vi "AFMss_control_DelayObserver_trajTrack.vi"() -> ()   [LabVIEW 2017]
uses:
  controls/controlParams_tracktraj.ctl
  controls/Xdelay.ctl
  <vilib>/rvi/Emulation/niFpgaGetClockAttributes.vi
  <vilib>/rvi/Emulation/niFpgaSctlEmulationGetInTimedLoop.vi
  <vilib>/rvi/Emulation/niFpgaEmulationReportErrorSimple.vi
  <vilib>/rvi/eio/common/nirviEmuTemplateMethod_errors.vi
  <vilib>/rvi/Emulation/niFpgaCriticalErrorInLSC.vi
  <vilib>/rvi/DataTransferAndStorage/Container/Common/niFpgaContainerExecOnDevCompGetState.vi
  <vilib>/rvi/Emulation/niFpgaEmulationIsFPGAContextNoSignature.vi
  <vilib>/rvi/DataTransferAndStorage/Container/Common/niFpgaContainerGetUniqueNameForEmu.vi
  <vilib>/rvi/Memory/Memory_Emulation/niFpgaMemoryEmulationCacheClearOnFirstRun.vi
  <vilib>/rvi/Memory/Memory_Emulation/nirvimemoryEmulationManagerCache_MakeExclusive.vi
  <vilib>/rvi/Memory/Memory_Emulation/niFpgaMemoryEmulationValidateCache.vi
  <vilib>/rvi/Memory/Memory_Emulation/nirvimemoryEmulationManagerCache_InsertValue.vi
  <vilib>/Utility/error.llb/Clear Errors.vi
  <vilib>/rvi/Memory/Memory_Emulation/nirvimemoryEmulationManagerCache_ReleaseExclusive.vi
  <vilib>/rvi/Memory/Memory_Emulation/nirvimemoryEmulationManagerCache_GetValue.vi
  <vilib>/rvi/Memory/Memory_Emulation/nirvimemoryEmulationManagerCache_SetValue.vi
  <vilib>/rvi/Emulation/niFpgaProcessEmulError.vi
  <vilib>/rvi/interface/RandomDataEmulation/niFpgaRandomDataHandleErrors.vi
  <vilib>/eio/EIONode/EIONode.xnode
  <vilib>/rvi/DataTransferAndStorage/Container/XNode/niFpgaContainer.xnode
  <vilib>/rvi/DataTransferAndStorage/Register/Emulation/niFpgaRegisterEmulationRefIn.vi
  <vilib>/rvi/interface/RandomDataEmulation/nirviRandomDataFpgaReadWriteTemplate.vi
  <vilib>/rvi/FXPMathLib/FxpSub/XNode/nifxpmath_Sub.xnode
  <vilib>/rvi/FXPMathLib/sim/FxpSim.dll
panel:
  out "Xd_out(k+1)":T1
  out "yk":sgl
  out "u_xk":sgl
  out "yuxk TO":bool
  out "YK TO":bool
  out "UK TO":bool
  in  "Cluster":T2={"umax"=3.0, "y_ref(k)"=0.0, "Ki"=0.0, "y(k) (from plant)"=0.0, "ND"=0, "NS"=0, "u_Kx_ref(k)"=0.0} {"u_Kx_ref(k)" format="%#_13g"; "Ki" format="%#_13g"; "y_ref(k)" format="%#_13g"; "umax" format="%#_13g"}
  out "Unstable Traj":bool
  out "ND":i16=2
  out "Loop Done":bool
  in  "Settle Ticks":i16=1000
  in  "False  = cont run":bool=TRUE
  in  "Abort":bool=TRUE
  in  "iters":i16=1
  in  "ymax":sgl=4.0 format="%#_13g"
  in  "TsTicks":i16
  out "Loop Ticks (benchmark)":i16
  out "NS":i16=2
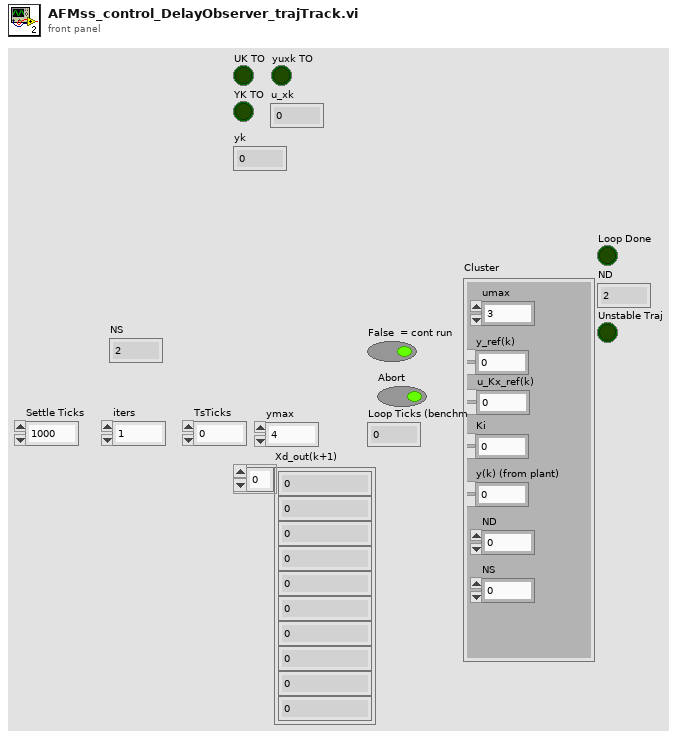
[diagram p1: front panel]
types:
  T1 = typedef "Xdelay.ctl" = sgl[]
  T2 = typedef "controlParams_tracktraj.ctl" = cluster{"umax":sgl, "y_ref(k)":sgl, "Ki":sgl, "y(k) (from plant)":sgl, "ND":i16, "NS":i16, "u_Kx_ref(k)":sgl}
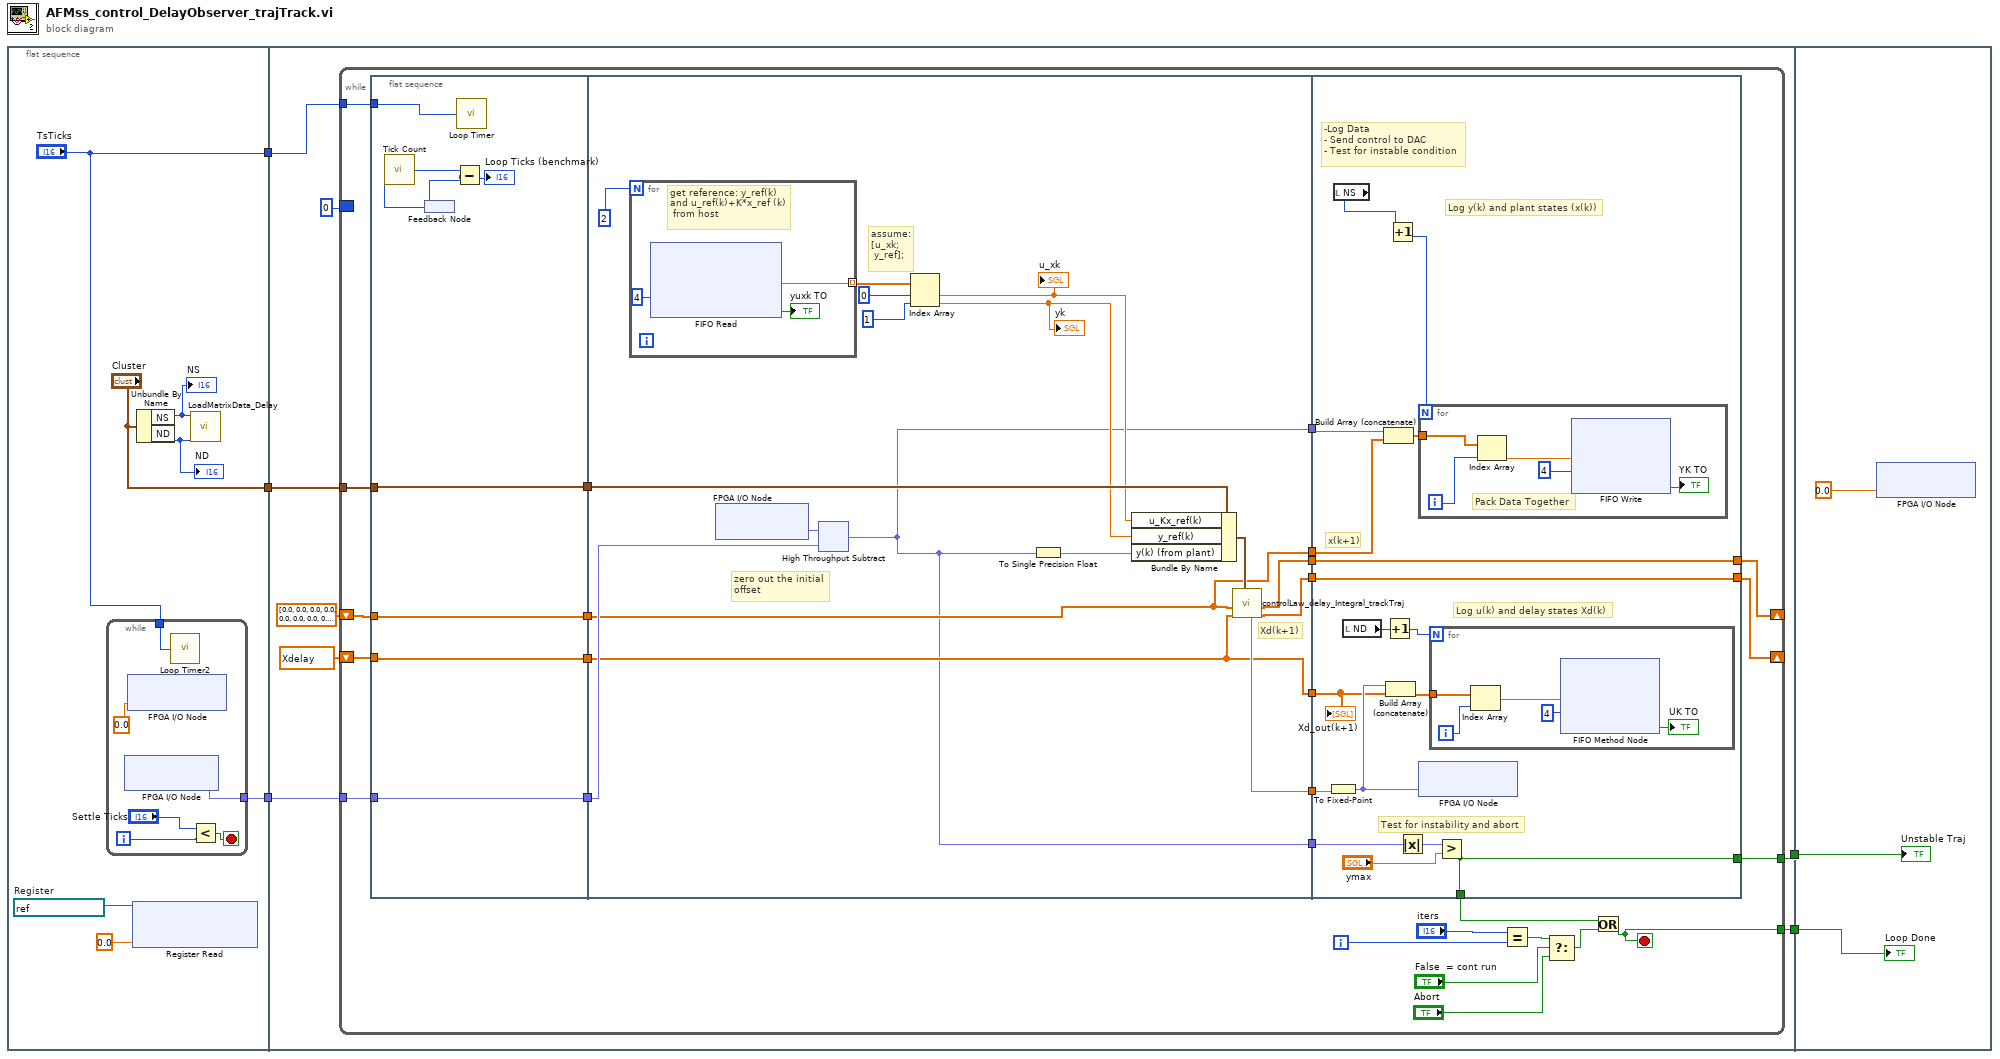
[diagram p0: block diagram]
diagram:
  n1 = flat-sequence {
    tunnel: ["TsTicks"] -> w5
    tunnel: [w12] -> w4
    tunnel: ["Cluster"] -> w2
    tunnel: w5 -> [w25]
    tunnel: w4 -> [w24]
    tunnel: [w21] -> w3
    tunnel: w2 -> [w20]
    tunnel: [w19] -> w1
    tunnel: w3 -> [w110]
    tunnel: w1 -> [w109]
    frame #0 {
      w10 = refnum<k21> "accumulator"  # Register
      # "Load Matrix Data"
      n2 = while {
        tunnel: [w18] -> w12
        tunnel: "TsTicks" -> [w17]
        i -> [w13]
        stop <- w15 stop-if-true
        n3 = xnode "FPGA I/O Node"() -> ("Mod2/AI0"=w18:fxp<+/-,24,5>)  [unwired: 1 in, 1 out]
        n4 = xnode "FPGA I/O Node"("Mod1/AO0"=sgl 0.0) -> ()  [unwired: 1 in, 1 out]
        n5 = call "Loop Timer2"("Count(Ticks)"=w17) -> ()  [unwired: 1 out]
        n6 = Less?(x="Settle Ticks", y=w13) -> (x < y?=w15:bool)
      }
      n7 = xnode ("Register Read")("Data"=sgl 0.0, "Register In"=w10) -> ()  [unwired: 1 out]
      n8 = Unbundle By Name("Cluster") -> ("NS"=w8:i16, "ND"=w7:i16)
      "NS" <- w8
      "ND" <- w7
      n9 = call "LoadMatrixData_Delay.vi"("Nd"=w7, "NS"=w8) -> ()  [unwired: 9 in, 1 out]
    }
    frame #1 {
      n10 = while {
        border: i16 0 -> [_]
        tunnel: w25 -> [w44]
        tunnel: w24 -> [w42]
        shift-right: [w36] -> _
        shift-left: T1 [0.0, 0.0, 0.0, 0.0, 0.0, 0.0, 0.0, 0.0, 0.0, 0.0, 0.0, 0.0] ("Xd_out(k+1)") -> [w35]
        shift-right: [w30] -> _
        shift-left: sgl[] [0.0, 0.0, 0.0, 0.0, 0.0, 0.0, 0.0, 0.0, 0.0, 0.0, 0.0, 0.0, 0.0, 0.0, 0.0, 0.0, 0.0, 0.0, 0.0, 0.0, 0.0, 0.0, 0.0, 0.0, 0.0] ("x^(k+1) = Ax + Bu + Lye") -> [w39]
        tunnel: [w34] -> w21
        tunnel: w20 -> [w32]
        tunnel: [w31] -> w19
        i -> [w49]
        stop <- w34 stop-if-true
        n11 = flat-sequence {
          tunnel: w44 -> [w58]
          tunnel: w42 -> [w57]
          tunnel: [w57] -> w41
          tunnel: [w55] -> w40
          tunnel: w39 -> [w56]
          tunnel: [w56] -> w38
          tunnel: w35 -> [w55]
          tunnel: [w54] -> w33
          tunnel: w32 -> [w54]
          tunnel: [w72] -> w53
          tunnel: [w73] -> w52
          tunnel: [w62] -> w43
          tunnel: w41 -> [w78]
          tunnel: w40 -> [w64]
          tunnel: w38 -> [w63]
          tunnel: [w71] -> w37
          tunnel: w33 -> [w75]
          tunnel: [w64] -> w29
          tunnel: [w63] -> w28
          tunnel: [w62] -> w27
          tunnel: w53 -> [w84]
          tunnel: w52 -> [w91]
          tunnel: [w86] -> w51
          tunnel: w43 -> [w95]
          tunnel: w37 -> [w90]
          tunnel: [w90] -> w36
          tunnel: [w86] -> w31
          tunnel: [w84] -> w30
          tunnel: w29 -> [w85]
          tunnel: w28 -> [w83]
          tunnel: w27 -> [w82]
          frame #0 {
            n12 = call "Tick Count"() -> ("Tick Count(Ticks)"=w59:u32)
            n13 = feedback #1() -> (w60:u32)
            n14 = feedback-in #1(w59) -> ()
            n15 = Subtract(x=w59, y=w60) -> (x-y=→"Loop Ticks (benchmark)":u32)
            n16 = call "Loop Timer"("Count(Ticks)"=w58) -> ()  [unwired: 1 out]
          }
          frame #1 {
            # "assume:\n[u_xk;\n y_ref];"
            # "Xd(k+1)"
            # "zero out the initial \noffset"
            n17 = for {
              N: i16 2 -> [_]
              tunnel: [w80] -> w69 mode=indexing
              # "get reference: y_ref(k)\nand u_ref(k)+K*x_ref (k)\n from host"
              n18 = xnode ("FIFO Read")("Timeout"=i16 4) -> ("Element"=w80:sgl, "Timed Out?"=→"yuxk TO":bool)  [unwired: 1 in, 1 out]
            }
            n19 = xnode "FPGA I/O Node"() -> ("Mod2/AI0"=w77:fxp<+/-,24,5>)  [unwired: 1 in, 1 out]
            n20 = xnode "High Throughput Subtract"("x"=w77, "y"=w78) -> ("x-y"=w62:fxp<+/-,40,6>)
            n21 = Index Array(array=w69, index #1=i16 0, index #2=i16 1) -> (element #1=w66:sgl, element #2=w65:sgl)
            "u_xk" <- w66
            "yk" <- w65
            n22 = To Single Precision Float(number=w62) -> (single precision float=w76:sgl)
            n23 = Bundle By Name(cluster=w75, "u_Kx_ref(k)"=w66, "y_ref(k)"=w65, "y(k) (from plant)"=w76) -> (w74:T2)
            n24 = call "controlLaw_delay_Integral_trackTraj.vi"("Cluster"=w74, "Xd_in"=w64, "x^(k)"=w63) -> ("Xd_out(k+1)"=w71:T1, "x^(k+1) = Ax + Bu + Lye"=w72:sgl[], "u(k) (saturated)"=w73:sgl)  [unwired: 6 in]
          }
          frame #2 {
            # "x(k+1)"
            # "Log u(k) and delay states Xd(k)"
            # "Log y(k) and plant states (x(k))"
            # "-Log Data\n- Send control to DAC\n- Test for instable condition"
            # "Test for instability and abort"
            n25 = To Fixed-Point(number=w91) -> (fixed-point=w87:fxp<+/-,32,6>)  [unwired: 1 in]
            n26 = local read "NS"() -> (w92:i16)
            n27 = local read "ND"() -> (w94:i16)
            n28 = Build Array (concatenate)(w95, w83) -> (w96:sgl[])
            n29 = Increment(x=w94) -> (x+1=w88:i16)
            n30 = Build Array (concatenate)(w87, w85) -> (w89:sgl[])
            n31 = Increment(x=w92) -> (x+1=w93:i16)
            n32 = Absolute Value(x=w82) -> (abs(x)=w98:fxp<+,40,6>)
            n33 = for {
              N: w93 -> [_]
              tunnel: w96 -> [w106]
              i -> [w107]
              # "Pack Data Together"
              n34 = Index Array(array=w106, index=w107) -> (element=w105:sgl)
              n35 = xnode ("FIFO Write")("Element"=w105, "Timeout"=i16 4) -> ("Timed Out?"=→"YK TO":bool)  [unwired: 1 in, 1 out]
            }
            n36 = xnode "FPGA I/O Node"("Mod1/AO0"=w87) -> ()  [unwired: 1 in, 1 out]
            n37 = for {
              N: w88 -> [_]
              tunnel: w89 -> [w100]
              i -> [w102]
              n38 = Index Array(array=w100, index=w102) -> (element=w101:sgl)
              n39 = xnode ("FIFO Method Node")("Element"=w101, "Timeout"=i16 4) -> ("Timed Out?"=→"UK TO":bool)  [unwired: 1 in, 1 out]
            }
            n40 = Greater?(x=w98, y="ymax") -> (0:w86:bool)
            "Xd_out(k+1)" <- w85
          }
        }
        n41 = Equal?(x="iters", y=w49) -> (x = y?=w47:bool)
        n42 = Select(t=w47, s="False  = cont run", f="Abort") -> (s? t:f=w48:bool)
        n43 = Or(x=w51, y=w48) -> (x .or. y?=w34:bool)
      }
    }
    frame #2 {
      n44 = xnode "FPGA I/O Node"("Mod1/AO0"=sgl 0.0) -> ()  [unwired: 1 in, 1 out]
      "Loop Done" <- w110
      "Unstable Traj" <- w109
    }
  }
